vi "mkfifo.vi"(8 "error in (no error)":errorcluster, 10 "permissions (664)":T1={"owner"={"read"=TRUE, "write"=TRUE, "execute"=FALSE}, "group"={"read"=TRUE, "write"=TRUE, "execute"=FALSE}, "everyone"={"read"=TRUE, "write"=FALSE, "execute"=FALSE}}, 11 "pathname in":string) -> (0 "error out":errorcluster, 3 "pathname out":string)   [LabVIEW 2013, in "Linux RT IPC.C.lvlib"]
uses:
  Linux RT IPC.C.lvlib
  Controls/functions.ctl
  <vilib>/NI/NI Linux RT Errno/Linux Errno.lvlib
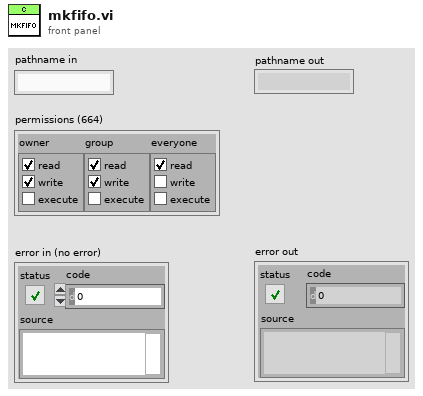
[diagram p1: front panel]
types:
  T1 = cluster{"owner":cluster{"read":bool, "write":bool, "execute":bool}, "group":cluster{"read":bool, "write":bool, "execute":bool}, "everyone":cluster{"read":bool, "write":bool, "execute":bool}}
  T2 = typedef "Linux RT IPC.C.lvlib/functions.ctl" = enum16{"unspecified", "close", "fstat", "ftruncate", "mkfifo", "mmap", "munmap", "open", "read", "shm_open", "shm_unlink", "write", "unlink"}
  T3 = typedef "Linux Errno.lvlib/errno.ctl" = enum16{"NO ERROR", "EPERM", "ENOENT", "ESRCH", "EINTR", "EIO", "ENXIO", "E2BIG", "ENOEXEC", "EBADF", "ECHILD", "EAGAIN", "ENOMEM", "EACCES", "EFAULT", "ENOTBLK", "EBUSY", "EEXIST", "EXDEV", "ENODEV", "ENOTDIR", "EISDIR", "EINVAL", "ENFILE", "EMFILE", "ENOTTY", "ETXTBSY", "EFBIG", "ENOSPC", "ESPIPE", "EROFS", "EMLINK", "EPIPE", "EDOM", "ERANGE", "EDADLK", "ENAMETOOLONG", "ENOLCK", "ENOSYS", "ENOTEMPTY", "ELOOP", "EWOULDBLOCK", "ENOMSG", "EIDRM", "ECHRNG", "EL2NSYNC", "EL3HLT", "EL3RST", "ELNRNG", "EUNATCH", "ENOCSI", "EL2HLT", "EBADE", "EBADR", "EXFULL", "ENOANO", "EBADRQC", "EBADSLT", "EDEADLOCK", "EBFONT", "ENOSTR", "ENODATA", "ETIME", "ENOSR", "ENONET", "ENOPKG", "EREMOTE", "ENOLINK", "EADV", "ESRMNT", "ECOMM", "EPROTO", "EMULTIHOP", "EDOTDOT", "EBADMSG", "EOVERFLOW", "ENOTUNIQ", "EBADFD", "EREMCHG", "ELIBACC", "ELIBBAD", "ELIBSCN", "ELIBMAX", "ELIBEXEC", "ELISEQ", "ERESTART", "ESTRPIPE", "EUSERS", "ENOTSOCK", "EDESTADDRREQ", "EMSGSIZE", "EPROTOTYPE", "ENOPROTOOPT", "EPROTONOSUPPORT", "ESOCKTNOSUPPORT", "EOPNOTSUPP", "EPFNOSUPPORT", "EAFNOSUPPORT", "EADDRINUSE", "EADDRNOTAVAIL", "ENETDOWN", "ENETUNREACH", "ENETRESET", "ECONNABORTED", "ECONNRESET", "ENOBUFS", "EISCONN", "ENOTCONN", "ESHUTDOWN", "ETOOMANYREFS", "ETIMEDOUT", "ECONNREFUSED", "EHOSTDOWN", "EHOSTUNREACH", "EALREADY", "EINPROGRESS", "ESTALE", "EUCLEAN", "ENOTNAM", "ENAVAIL", "EISNAM", "EREMOTEIO", "EDQUOT", "ENOMEDIUM", "EMEDIUMTYPE", "ECANCELED", "ENOKEY", "EKEYEXPIRED", "EKEYREVOKED", "EKEYREJECTED", "EOWNERDEAD", "ENOTRECOVERABLE", "ERFKILL", "EHWPOISON", "UNDEFINED"}
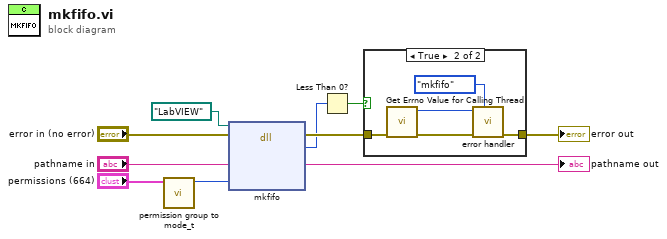
[diagram p0: block diagram]
diagram:
  n1 = call "permission group to mode_t.vi"("permissions group"="permissions (664)") -> ("mode_t"=w7:u32)  [unwired: 10 in]
  n2 = dll-call lib="LabVIEW" fn="mkfifo"(path in=path "LabVIEW", error in="error in (no error)", "pathname"="pathname in", "mode"=w7) -> (error out=w5:errorcluster, "return"=w2:i32, "pathname"=→"pathname out":string)  [unwired: 2 in, 1 out]
  n3 = Less Than 0?(x=w2) -> (x < 0?=w4:bool)
  n4 = case shown="True" w4 {
    tunnel: w5 -> [w11 w16]
    tunnel: [w11 w15] -> w3
    frame False {
    }
    frame True {
      n5 = call <vilib>:"Get Errno Value for Calling Thread.vi"("error in (no error)"=w16) -> ("error out"=w13:errorcluster, "errno"=w14:T3)  [unwired: 9 in]
      n6 = call "error handler.vi"("function (unspecified)"=functions."mkfifo" ("function"), "error in (no error)"=w13, "errno"=w14) -> ("error out"=w15:errorcluster)  [unwired: 8 in]
    }
  }
  "error out" <- w3
